vi "Fetch Data from Server.vi"(2 "error IN":errorcluster, 4 "query string":string="SELECT * FROM dbo.ThreatCalibers") -> (0 "error OUT":errorcluster, 1 "recordset data":string[][](array[string]))   [LabVIEW 2010]
uses:
  <vilib>/addons/database/Connection.llb/DB Tools Open Connec (Path).vi
  <vilib>/addons/database/Connection.llb/Conn Execute.vi
  <vilib>/addons/database/Recordset.llb/Rec Destroy - Connection.vi
  <vilib>/addons/database/NI_Database_API.lvlib
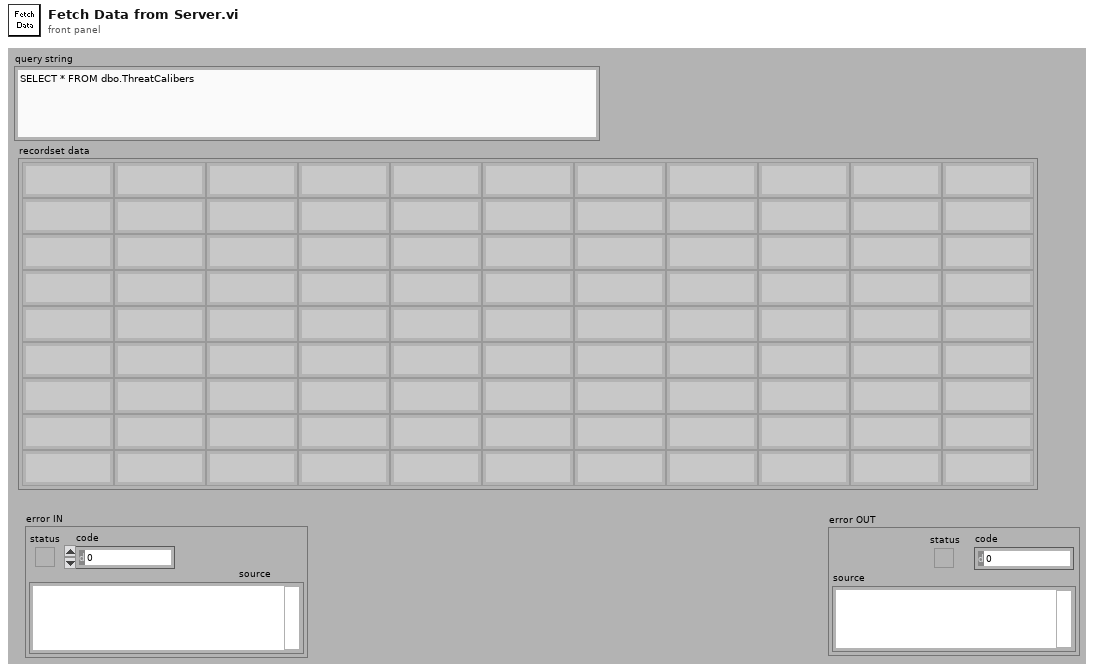
[diagram p1: front panel]
types:
  T1 = typedef "NI_Database_API.lvlib/Conn ObjectReference.ctl" = refnum<k1>
  T2 = typedef "NI_Database_API.lvlib/Rec ObjectReference.ctl" = refnum<k1>
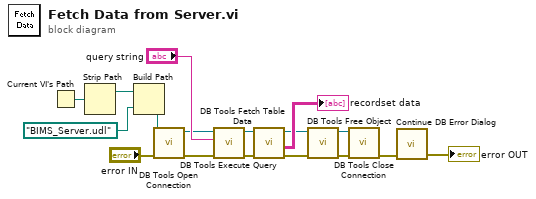
[diagram p0: block diagram]
diagram:
  n1 = Current VI's Path() -> (path=w4:path)
  n2 = Strip Path(path=w4) -> (stripped path=w3:path)  [unwired: 1 out]
  n3 = Build Path(base path=w3, name or relative path=path "BIMS_Server.udl" ("connectString")) -> (appended path=w1:path)
  n4 = call-poly <vilib>:"DB Tools Open Connection.vi"("error in (no error)"="error IN", "connection information"=w1) -> ("error out"=w9:errorcluster, "connection reference"=w7:T1)  [unwired: 3 in, 3 out]
  n5 = call-poly <vilib>:"DB Tools Execute Query.vi"("error in (no error)"=w9, "SQL query"="query string", "connection reference"=w7) -> ("error out"=w10:errorcluster, "recordset reference"=w6:T2)  [unwired: 1 in, 4 out]
  n6 = call <vilib>:"DB Tools Fetch Table Data.vi"("error in (no error)"=w10, "recordset reference"=w6) -> ("error out"=w11:errorcluster, "recordset data"=→"recordset data":string[][], "recordset reference out"=w5:T2)  [unwired: 3 out]
  n7 = call-poly <vilib>:"DB Tools Free Object.vi"("error in (no error)"=w11, "recordset reference"=w5) -> ("error out"=w12:errorcluster, "connection reference"=w8:T1)  [unwired: 8 out]
  n8 = call <vilib>:"DB Tools Close Connection.vi"("error in (no error)"=w12, "connection reference"=w8) -> ("error out"=w15:errorcluster)  [unwired: 5 out]
  n9 = call "Continue DB Error Dialog.vi"("error in (no error)"=w15) -> ("error out"=→"error OUT":errorcluster)  [unwired: 3 in, 2 out]
